vi "速度模式.vi"(8 "error in (no error)":errorcluster, 9 "Reset Count":bool, 10 "Max Torque":sgl=9.0, 11 "Velocity":sgl=9.0) -> (0 "error out":errorcluster)   [LabVIEW 2020, in "输出轴伺服.lvlib"]
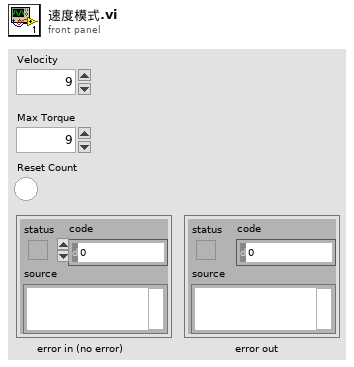
[diagram p1: front panel]
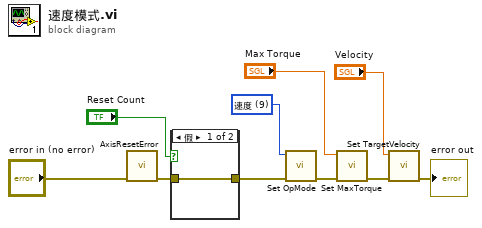
[diagram p0: block diagram]
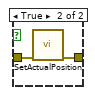
[diagram p2: hidden frame]
diagram:
  w1 = u32 9 items=["位置"=8, "速度"=9, "扭矩"=10] ("Value")
  n1 = call "AxisResetError.vi"("error in (no error)"="error in (no error)") -> ("error out"=w3:errorcluster)  [unwired: 10 in]
  n2 = case shown="假" "Reset Count" {
    tunnel: [w11 w13] -> w7
    tunnel: w3 -> [w11 w12]
    frame False {
    }
    frame True {
      n3 = call "SetActualPosition.vi"("error in (no error)"=w12) -> ("error out"=w13:errorcluster)  [unwired: 10 in]
    }
  }
  n4 = call "Set OpMode.vi"("error in (no error)"=w7, "Value"=w1) -> ("error out"=w2:errorcluster)  [unwired: 9 in]
  n5 = call "Set MaxTorque.vi"("error in (no error)"=w2, "Value"="Max Torque") -> ("error out"=w10:errorcluster)  [unwired: 9 in]
  n6 = call "Set TargetVelocity.vi"("error in (no error)"=w10, "Value"="Velocity") -> ("error out"=→"error out":errorcluster)  [unwired: 9 in]
